vi "MoveAbs.vi"(8 "error in (no error)":errorcluster, 11 "DMC_1000B in":refnum<class "DMC_1000B.lvclass">) -> (0 "error out":errorcluster, 3 "DMC_1000B out":refnum<class "DMC_1000B.lvclass">)   [LabVIEW 2019, in "DMC_1000B.lvclass"]
uses:
  DMC_1000B.lvclass
  LLB/Commonly VI/Main Glb.vi
  LLB/DMC1000B/Dmc1000/Dmc1000.lvlib
  LLB/Commonly VI.lvlib
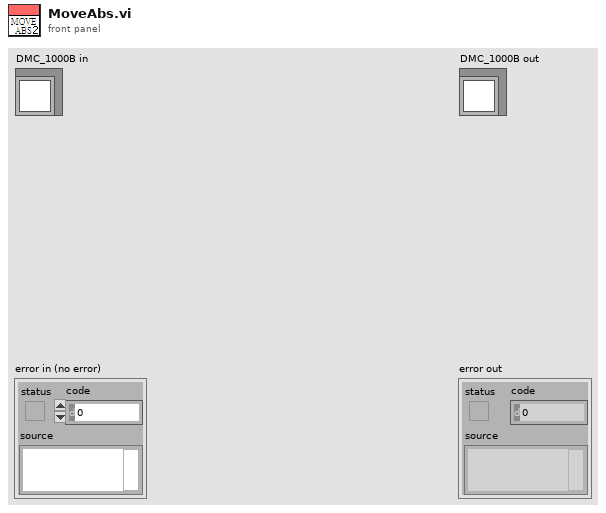
[diagram p1: front panel]
types:
  T1 = cluster{"AxisName":string, "Accel":dbl, "Deaccel":dbl, "Speed":dbl, "Sramp":dbl}[]
  T2 = cluster{"AxisName":string, "Accel":dbl, "Deaccel":dbl, "Speed":dbl, "Sramp":dbl}
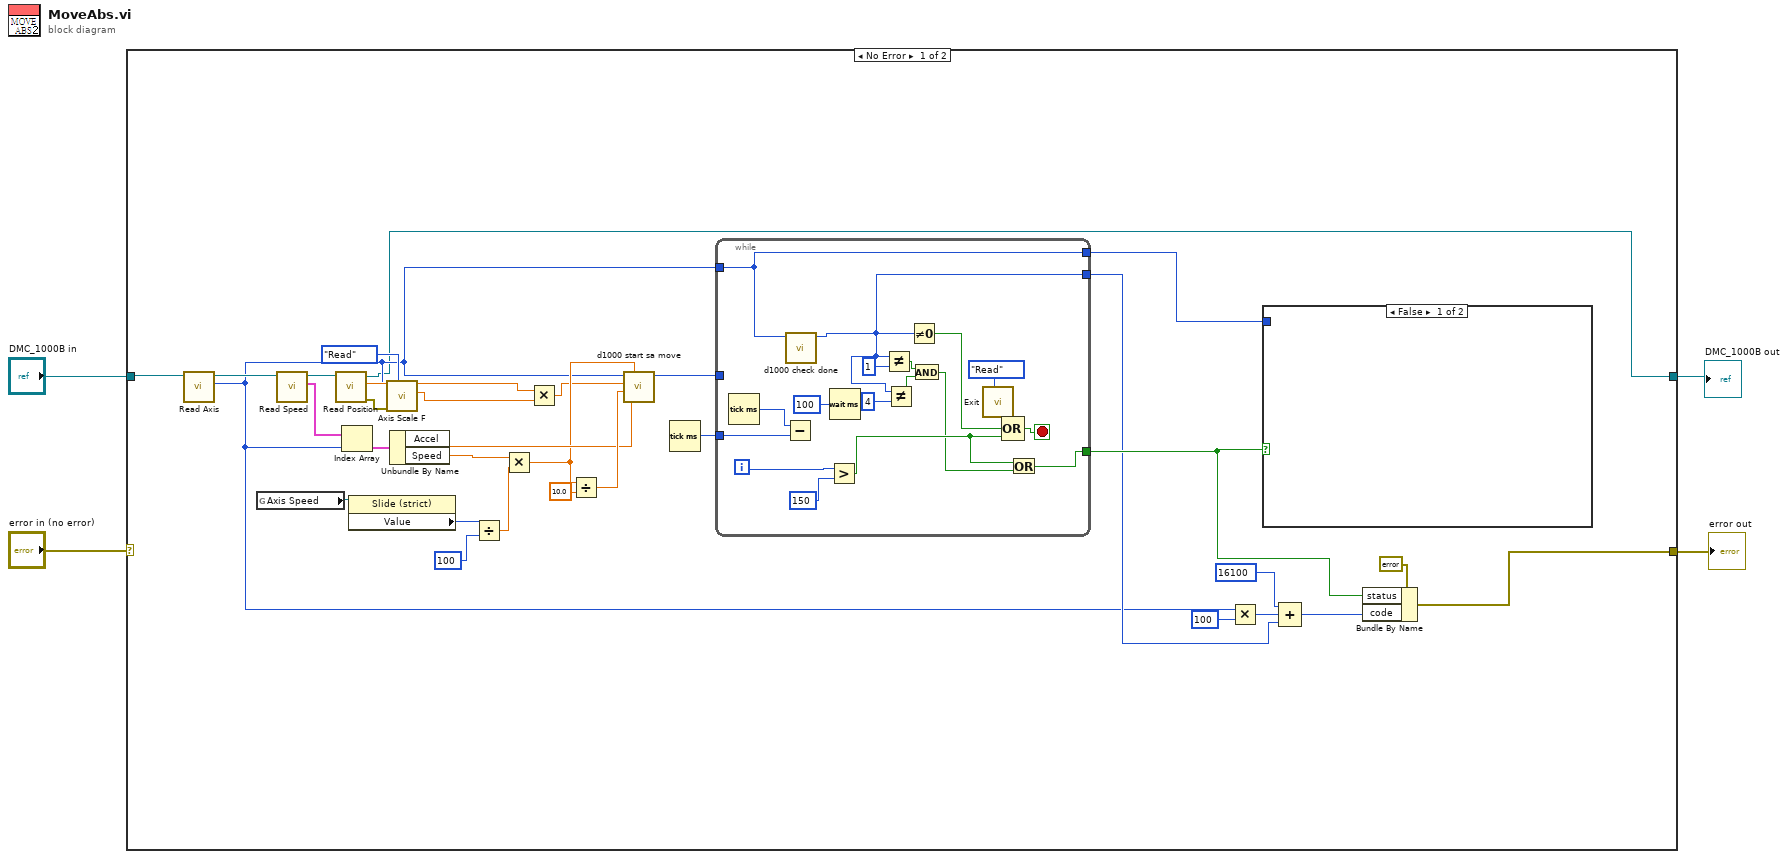
[diagram p0: block diagram]
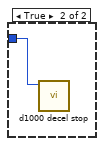
[diagram p2: hidden frame]
diagram:
  n1 = case shown="No Error" "error in (no error)" {
    selector: "error in (no error)" -> [_ w56]
    tunnel: "DMC_1000B in" -> [w24 w57]
    tunnel: [w5 w57] -> w2
    tunnel: [w22 w56] -> w1
    frame No Error {
      n2 = call-dynamic "Read Axis.vi"("AxisCard in"=w24) -> ("Axis"=w6:u32, "AxisCard out"=w36:refnum<class "DMC_1000B.lvclass">)  [unwired: 8 in, 1 out]
      n3 = global read "Main Glb.vi" "Axis Speed"() -> (w17:refnum<vi>)
      n4 = call-dynamic "Read Speed.vi"("AxisCard in"=w36) -> ("AxisSpeed"=w35:T1, "AxisCard out"=w23:refnum<class "DMC_1000B.lvclass">)  [unwired: 8 in, 1 out]
      n5 = call-dynamic "Read Position.vi"("AxisCard in"=w23) -> ("error out"=w11:errorcluster, "Position"=w10:dbl, "AxisCard out"=w5:refnum<class "DMC_1000B.lvclass">)  [unwired: 8 in]
      n6 = Index Array(array=w35, index=w6) -> (element=w34:T2)
      n7 = property class="Slide (strict)"(reference=w17) -> ("Value"=w16:i32)  [unwired: 1 in, 2 out]
      n8 = call "Axis Scale F.vi"("Enum"=enum16{"Initial", "Read"}."Read", "error In"=w11, "Axis"=w6) -> ("Scale"=w9:dbl)  [unwired: 7 in, 1 out]
      n9 = Unbundle By Name(w34) -> ("Accel"=w19:dbl, "Speed"=w14:dbl)
      n10 = Divide(x=w16, y=100) -> (x/y=w13:dbl)
      n11 = Multiply(x=w14, y=w13) -> (x*y=w12:dbl)
      n12 = Multiply(x=w10, y=w9) -> (x*y=w8:dbl)
      n13 = Divide(x=w12, y=10.0) -> (x/y=w21:dbl)
      n14 = call "d1000 start sa move.vi"("Tacc"=w19, "MaxVel"=w12, "StrVel"=w21, "Pos"=w8, "axis"=w6) -> ("function return"=w18:u32)  [unwired: 6 in]
      n15 = Tick Count (ms)() -> (millisecond timer value=w33:u32)
      n16 = while {
        tunnel: w6 -> [w51]
        tunnel: w33 -> [w53]
        tunnel: [w51] -> w32
        tunnel: [w48] -> w26
        tunnel: [w39] -> w25
        tunnel: w18 -> [_]
        i -> [w46]
        stop <- w49 stop-if-true
        n17 = Tick Count (ms)() -> (millisecond timer value=w54:u32)
        n18 = Subtract(x=w54, y=w53) -> ()  [unwired: 1 out]
        n19 = call "d1000 check done.vi"("axis"=w51) -> ("function return"=w39:u32)  [unwired: 10 in]
        n20 = Greater?(x=w46, y=u32 150) -> (0:w47:bool)
        n21 = Wait (ms)(milliseconds to wait=u32 100) -> ()  [unwired: 1 out]
        n22 = Not Equal?(x=w39, y=u32 1) -> (x != y?=w43:bool)
        n23 = Not Equal?(x=w39, y=u32 4) -> (x != y?=w40:bool)
        n24 = Not Equal To 0?(x=w39) -> (x != 0?=w38:bool)
        n25 = And(x=w43, y=w40) -> (x .and. y?=w41:bool)
        n26 = call "Exit.vi"("Enum"=enum16{"Initial", "Read", "Write"}."Read") -> ("ExitOut"=w45:bool)  [unwired: 10 in]
        n27 = Compound Arithmetic op=OR(w45, w38, w47) -> (w49:bool)
        n28 = Or(x=w47, y=w41) -> (x .or. y?=w48:bool)
      }
      n29 = Multiply(x=w6, y=u32 100) -> (x*y=w30:u32)
      n30 = case shown="False" w26 {
        tunnel: w32 -> [_ w37]
        frame False {
        }
        frame True {
          n31 = call "d1000 decel stop.vi"("axis"=w37) -> ()  [unwired: 10 in, 1 out]
        }
      }
      n32 = Compound Arithmetic op=ADD(16100, w30, w25) -> (w27:u32)
      n33 = Bundle By Name(cluster=errorcluster {"status"=FALSE, "code"=0, "source"=""} ("error constant"), "status"=w26, "code"=w27) -> (w22:errorcluster)
    }
    frame Error {
    }
  }
  "error out" <- w1
  "DMC_1000B out" <- w2
